vi "Data Collect2.vi"(0 "Data":string[](array[string]), 1 "Motion Postion List":string[][](table)=[["16537", "0", "0", "0"], ["16537", "0", "0", "0"], ["38723", "0", "0", "0"], ["Null", "Null", "Null", "Null"], ["Null", "Null", "Null", "Null"]], 2 "XY轴系数":string[][](array[string]), 3 "9点校正参数":string[][](table)=[["Null", "Null", "Null", "Null"], ["Null", "Null", "Null", "Null"], ["Null", "Null", "Null", "Null"], ["Null", "Null", "Null", "Null"], ["Null", "Null", "Null", "Null"]], 4 "Radio":string="0.0046430644225189", 5 "Axis":string="0.002", 7 "offset":string[](array[string])) -> (14 "结果数组":T1, 15 "单次结果数据":string[](array[string]))   [LabVIEW 2015]
panel:
  out "Distances Y mm":dbl
  out "Distances X mm":dbl
  out "结果数组":dbl[][](array[numeric])
  out "Y向距离":string
  out "X向距离":string
  out "0.85孔径":string
  out "孔径":string
  # "44.85"
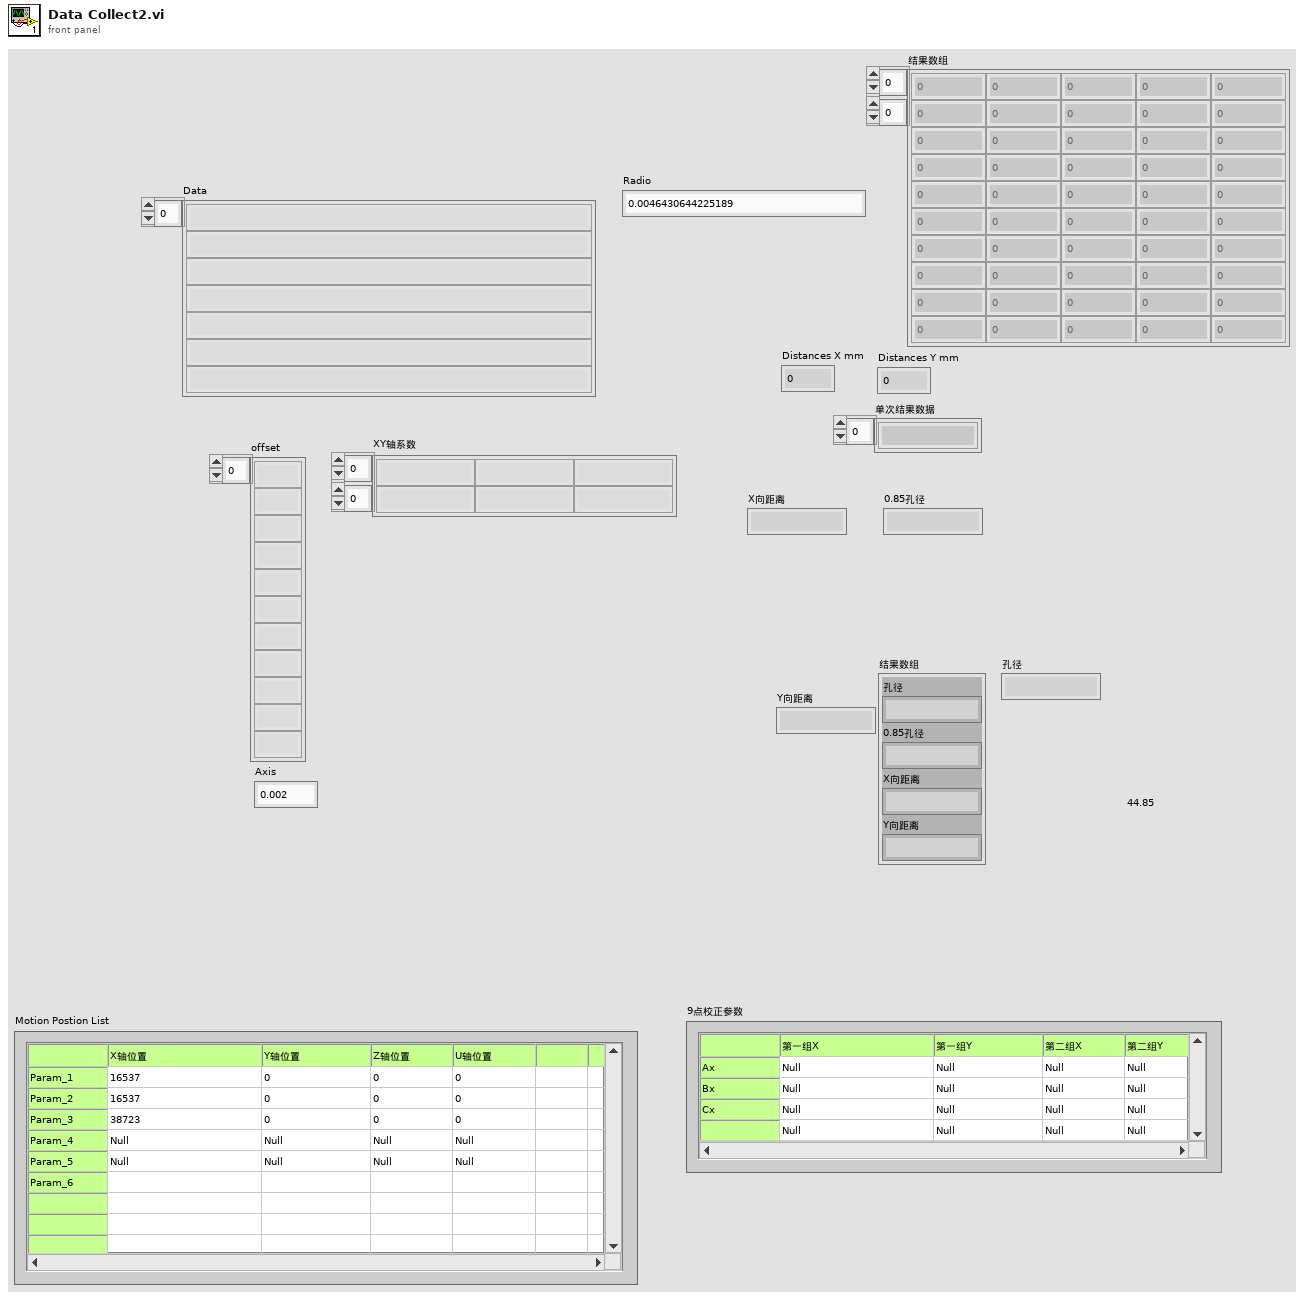
[diagram p1: front panel]
types:
  T1 = cluster{"孔径":string, "0.85孔径":string, "X向距离":string, "Y向距离 ":string}
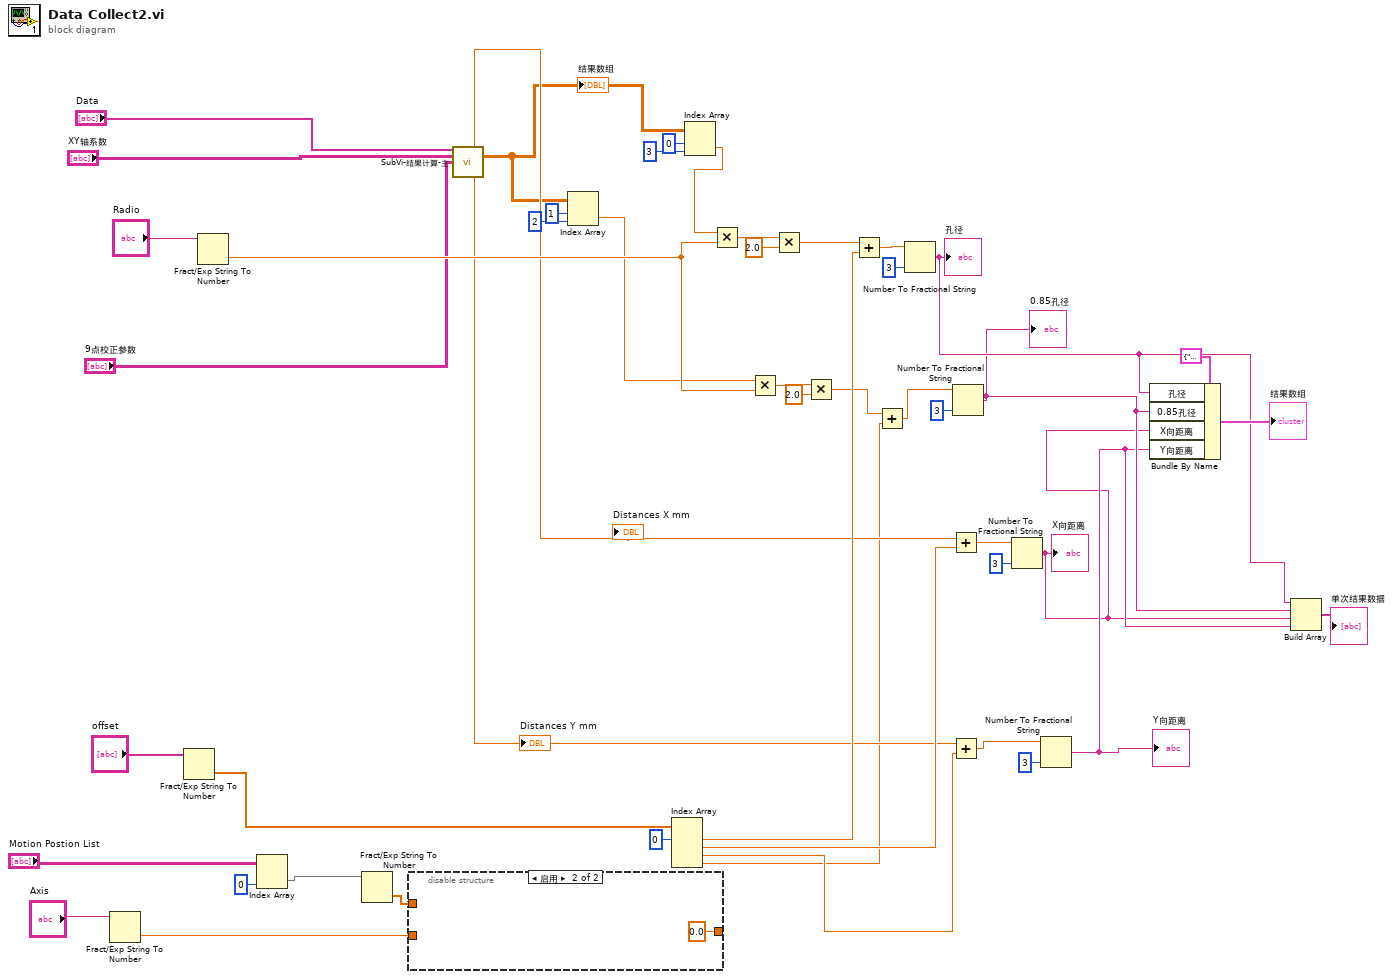
[diagram p0: block diagram]
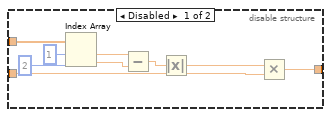
[diagram p2: hidden frame]
diagram:
  n1 = Fract/Exp String To Number(string="Axis") -> (number=w39:dbl)  [unwired: 3 in, 1 out]
  n2 = Fract/Exp String To Number(string="offset") -> (number=w37:dbl[])  [unwired: 3 in, 1 out]
  n3 = Fract/Exp String To Number(string="Radio") -> (number=w29:dbl)  [unwired: 3 in, 1 out]
  n4 = Index Array(array="Motion Postion List", index (col)=0 ("禁用的索引 (列)")) -> (element=w42:string[])  [unwired: 1 in]
  n5 = Fract/Exp String To Number(string=w42) -> (number=w41:dbl[])  [unwired: 3 in, 1 out]
  n6 = disable-structure shown="启用" {
    disable-tunnel: w41 -> [w57 _]
    disable-tunnel: w39 -> [w51 _]
    disable-tunnel: [w49 0.0] -> _
    frame Disabled {
      n7 = Index Array(array=w57, index #1=1 ("索引"), index #2=2 ("索引")) -> (element #1=w54:dbl, element #2=w53:dbl)
      n8 = Subtract(x=w54, y=w53) -> (x-y=w52:dbl)
      n9 = Absolute Value(x=w52) -> (abs(x)=w50:dbl)
      n10 = Multiply(x=w50, y=w51) -> (x*y=w49:dbl)
    }
    frame Enabled {
    }
  }
  n11 = call "SubVi-结果计算-主.vi"("图像处理的结果字符串"="Data", "XY轴系数"="XY轴系数", "9点校正参数"="9点校正参数") -> ("Distances X mm"=w14:dbl, "结果数组"=w3:dbl[][], "Distances Y mm"=w13:dbl)  [unwired: 9 in, 1 out]
  "结果数组" <- w3
  "Distances X mm" <- w14
  "Distances Y mm" <- w13
  n12 = Index Array(array=w3, index (row)=1 ("索引"), index (col)=2 ("禁用的索引 (列)")) -> (element=w1:dbl)
  n13 = Index Array(array=w37, index #1=0 ("索引")) -> (element #1=w31:dbl, element #2=w27:dbl, element #3=w11:dbl, element #4=w7:dbl)  [unwired: 3 in]
  n14 = Index Array(array=w3, index (row)=0 ("索引 (行)"), index (col)=3 ("禁用的索引 (列)")) -> (element=w8:dbl)
  n15 = Multiply(x=w8, y=w29) -> (x*y=w46:dbl)
  n16 = Multiply(x=w1, y=w29) -> (x*y=w33:dbl)
  n17 = Multiply(x=w46, y=2.0) -> (x*y=w30:dbl)
  n18 = Multiply(x=w33, y=2.0) -> (x*y=w6:dbl)
  n19 = Add(x=w30, y=w31) -> (x+y=w35:dbl)
  n20 = Add(x=w6, y=w7) -> (x+y=w5:dbl)
  n21 = Number To Fractional String(number=w35, precision (6)=i16 3 ("精度(6)")) -> (F-format string=w17:string)  [unwired: 2 in]
  "孔径" <- w17
  n22 = Add(x=w14, y=w27) -> (x+y=w26:dbl)
  n23 = Add(x=w13, y=w11) -> (x+y=w24:dbl)
  n24 = Number To Fractional String(number=w5, precision (6)=i16 3 ("精度(6)")) -> (F-format string=w16:string)  [unwired: 2 in]
  "0.85孔径" <- w16
  n25 = Number To Fractional String(number=w26, precision (6)=i16 3 ("精度(6)")) -> (F-format string=w12:string)  [unwired: 2 in]
  "X向距离" <- w12
  n26 = Number To Fractional String(number=w24, precision (6)=i16 3 ("精度(6)")) -> (F-format string=w15:string)  [unwired: 2 in]
  "Y向距离" <- w15
  n27 = Bundle By Name(cluster=T1 {"孔径"="", "0.85孔径"="", "X向距离"="", "Y向距离 "=""} ("输入簇"), "孔径"=w17, "0.85孔径"=w16, "X向距离"=w12, "Y向距离"=w15) -> (→"结果数组":T1)
  n28 = Build Array(w17, w16, w12, w15) -> (→"单次结果数据":string[])
